vi "Day 7 Puzzle 2.vi"() -> ()   [LabVIEW 2021]
panel:
  out "min value":i32
  out "How much space we need":i32
  out "Current space \navailable":i32
  out "Top dir size":i32
  out "Current set":cluster{string, i32}[](array[cluster])
  in  "Path":path
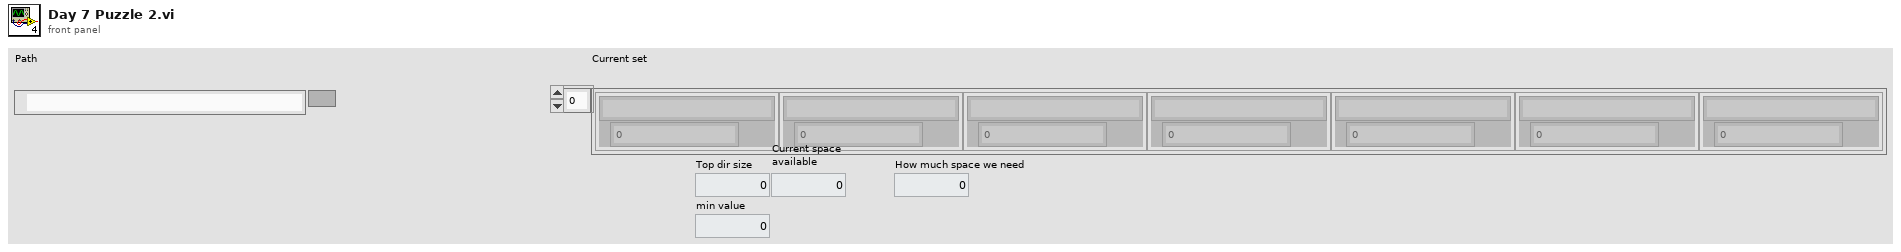
[diagram p1: front panel]
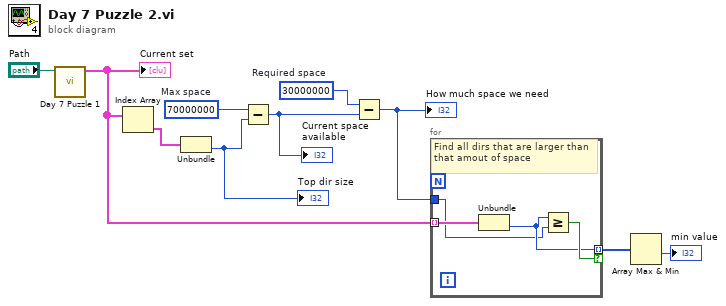
[diagram p0: block diagram]
diagram:
  w6 = 30000000  # Required space
  w7 = 70000000  # Max space
  n1 = call "Day 7 Puzzle 1.vi"("Path"="Path") -> ("Array"=w4:cluster{string, i32}[])  [unwired: 10 in]
  "Current set" <- w4
  n2 = Index Array(array=w4) -> (element=w9:cluster{string, i32})  [unwired: 1 in]
  n3 = Unbundle(w9) -> (w8:i32)  [unwired: 1 out]
  "Top dir size" <- w8
  n4 = Subtract(x=w7, y=w8) -> (x-y=w5:i32)
  "Current space \navailable" <- w5
  n5 = Subtract(x=w6, y=w5) -> (x-y=w3:i32)
  "How much space we need" <- w3
  n6 = for {
    tunnel: w4 -> [w14] mode=indexing
    tunnel: w3 -> [w11]
    tunnel: [w12] -> w2 mode=indexing if=w13
    # "Find all dirs that are larger than that amout of space"
    n7 = Unbundle(w14) -> (w12:i32)  [unwired: 1 out]
    n8 = Greater Or Equal?(x=w12, y=w11) -> (x >= y?=w13:bool)
  }
  n9 = Array Max & Min(array=w2) -> (min value=→"min value":i32)  [unwired: 3 out]
